vi "PATCH (File).vi"(6 "timeout":i32=10000, 7 "output file":path, 8 "error in":errorcluster, 9 "file":path, 10 "url":string, 11 "session in":refnum<class "Session.lvclass">) -> (0 "error out":errorcluster, 1 "body":string, 2 "headers":string, 3 "session out":refnum<class "Session.lvclass">, 4 "status code":u32)   [LabVIEW 2019, in "NI_Advanced HTTP Client.lvlib" / "Session.lvclass"]
uses:
  Session.lvclass
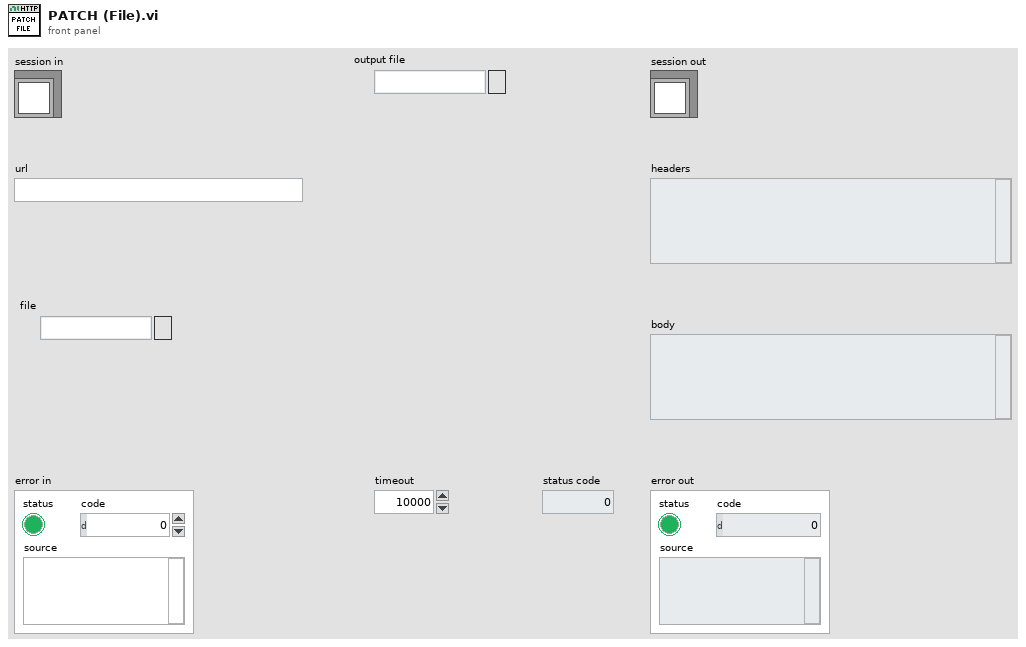
[diagram p1: front panel]
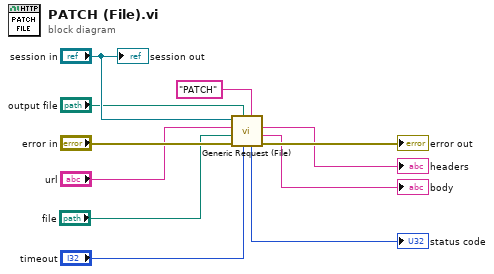
[diagram p0: block diagram]
diagram:
  n1 = call "Generic Request (File).vi"("method"="PATCH", "timeout"="timeout", "output file"="output file", "error in"="error in", "file"="file", "url"="url", "session in"="session in") -> ("error out"=→"error out":errorcluster, "body"=→"body":string, "headers"=→"headers":string, "status code"=→"status code":u32)  [unwired: 1 out]
  "session out" <- "session in"
